vi "NI9205_SUB-VI_INIT_OLD.vi"(8 "error in (no error)":errorcluster, 9 "Channels NI9205":tag, 10 "Number of Samples":i32, 11 "Sample Rate":dbl=1000.0) -> (0 "error out":errorcluster, 3 "Refnum out":refnum<k21>)   [LabVIEW 2020]
uses:
  <vilib>/DAQmx/create/channels.llb/DAQmx Create Channel (AI-Voltage-Basic).vi
  <vilib>/DAQmx/configure/timing.llb/DAQmx Timing (Sample Clock).vi
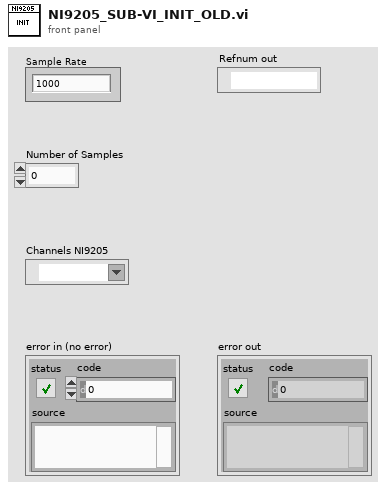
[diagram p1: front panel]
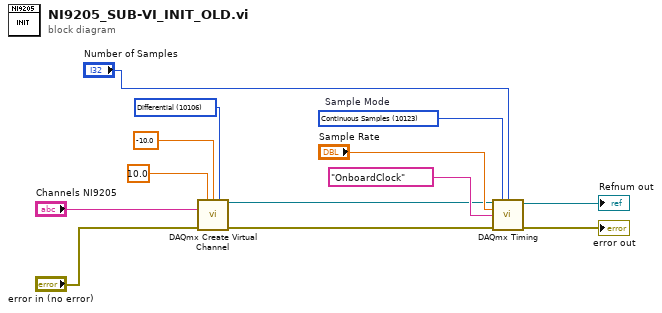
[diagram p0: block diagram]
diagram:
  w3 = 10106 items=["default"=-1, "RSE"=10083, "NRSE"=10078, "Differential"=10106, "Pseudodifferential"=12529] ("Terminal Configuration")
  w1 = 10123 items=["Finite Samples"=10178, "Continuous Samples"=10123, "Hardware Timed Single Point"=12522]  # Sample Mode
  n1 = call-poly <vilib>:"DAQmx Create Virtual Channel.vi"("maximum value"=10.0 ("Max Voltage"), "minimum value"=-10.0 ("Min Voltage"), "input terminal configuration"=w3, "physical channels"="Channels NI9205", "error in"="error in (no error)") -> ("task out"=w2:refnum<k21>, "error out"=w10:errorcluster)  [unwired: 9 in]
  n2 = call-poly <vilib>:"DAQmx Timing.vi"("task/channels in"=w2, "sample mode"=w1, "samples per channel"="Number of Samples", "rate"="Sample Rate", "source"=tag "OnboardClock" ("Sample Clock Source"), "error in"=w10) -> ("task out"=→"Refnum out":refnum<k21>, "error out"=→"error out":errorcluster)  [unwired: 8 in]
